vi "sensor allocate and open.vi"(11 "sensor_index":u32) -> (3 "function return":u32)   [LabVIEW 2019, in "apdm.lvlib"]
doc: "APDM_EXPORT apdm_device_handle_t apdm_sensor_allocate_and_open(const uint32_t sensor_index);"
uses:
  apdm.lvlib
  Lee Lab/CP FES Walking 2018/Code/Working/LabVIEW/apdm.dll
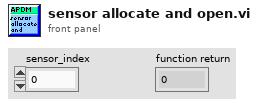
[diagram p1: front panel]
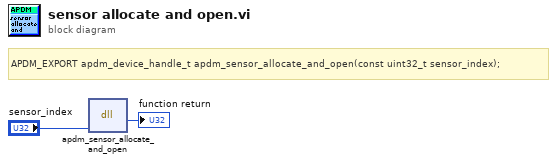
[diagram p0: block diagram]
diagram:
  # "APDM_EXPORT apdm_device_handle_t apdm_sensor_allocate_and_open(const uint32_t sensor_index);"
  n1 = dll-call lib="C:/Users/jfalesi/Dropbox/Lee Lab/CP FES Walking 2018/Code/Working/LabVIEW/apdm.*" fn="apdm_sensor_allocate_and_open"("sensor_index"="sensor_index") -> (→"function return":u32)  [unwired: 4 in, 2 out]
